vi "Read Settings.vi"(8 "error in":errorcluster) -> (0 "error out":errorcluster, 3 "No.Of Suggestions":i64)   [LabVIEW 2014, in "SmartPalette.lvlib"]
uses:
  SmartPalette.lvlib
  <vilib>/Utility/config.llb/Read Key (Double).vi
  <vilib>/Utility/config.llb/NI_LVConfig.lvlib
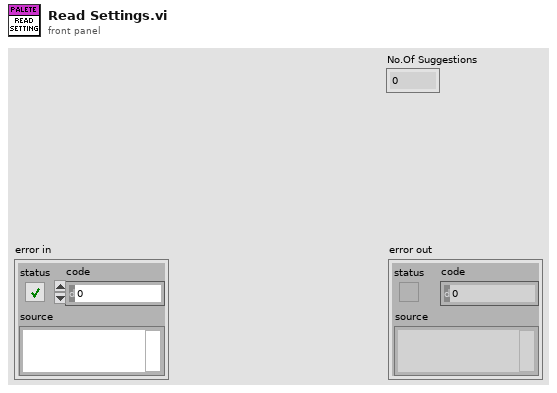
[diagram p1: front panel]
types:
  T1 = typedef "NI_LVConfig.lvlib/Config Data RefNum.ctl" = refnum<k1>
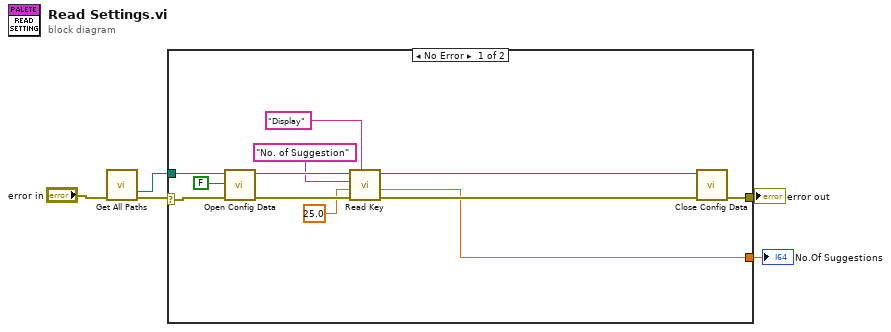
[diagram p0: block diagram]
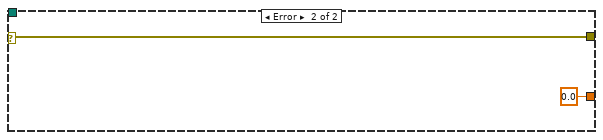
[diagram p2: hidden frame]
diagram:
  n1 = call "Get All Paths.vi"("error in"="error in") -> ("Smart Guider App file"=w5:path, "error out"=w4:errorcluster)  [unwired: 8 in, 5 out]
  n2 = case shown="No Error" w4 {
    selector: w4 -> [w9 w19]
    tunnel: w5 -> [w10 _]
    tunnel: [w8 w19] -> w2
    tunnel: [w6 0.0 ("value")] -> w1
    frame No Error {
      n3 = call <vilib>:"Open Config Data.vi"("error in (no error)"=w9, "create file if necessary (T)"=FALSE, "configuration file path"=w10) -> ("error out"=w16:errorcluster, "refnum"=w15:T1)  [unwired: 6 in, 1 out]
      n4 = call-poly <vilib>:"Read Key.vi"("section"="Display", "error in (no error)"=w16, "default value"=25.0, "key"="No. of Suggestion", "refnum"=w15) -> ("error out"=w14:errorcluster, "value"=w6:dbl, "refnum out"=w11:T1)  [unwired: 3 in, 1 out]
      n5 = call <vilib>:"Close Config Data.vi"("error in (no error)"=w14, "refnum"=w11) -> ("error out"=w8:errorcluster)  [unwired: 8 in, 1 out]
    }
    frame Error {
    }
  }
  "error out" <- w2
  "No.Of Suggestions" <- w1
